vi "Insight_Reduce_Data.vi"(6 "DV Threshold":dbl=0.5, 7 "Data Valid Type":enum16{"Software DV", "Hardware DV"}(ring), 8 "error in (no error)":errorcluster, 9 "Data Valid Data":dbl[](array[numeric]), 10 "Indices of Invalid Data":u32[](array[numeric]), 11 "Raw Data":dbl[](array[numeric])) -> (0 "error out":errorcluster, 3 "Processed Data":dbl[](array[numeric]))   [LabVIEW 2011]
doc: "This VI takes Raw data and the indices of invalid measurements and reduces it to Processed Data with only valid data.\n\nYou can reduce the data using either a \"Software Data Valid\" - a vector of the invalid points - or a \"Hardware Data Valid\" - which is a vector acquired simultaneous with the Raw Data. Use the Enum to select which type you are using and provide either the \"Indices of Invalid Data\" fot \"Software Data Valid\", or the \"Data Valid Data\" and \"DV Threshold\" for \"Hardware Data Valid\"."
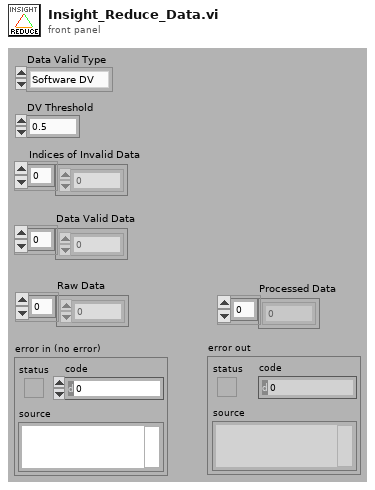
[diagram p1: front panel]
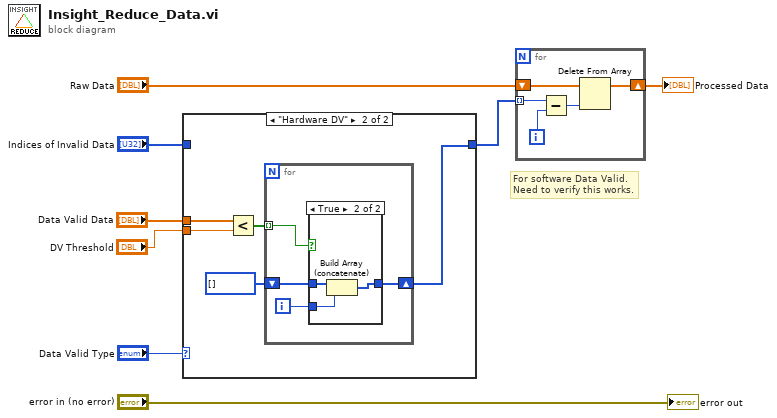
[diagram p0: block diagram]
diagram:
  # "For software Data Valid.\nNeed to verify this works."
  n1 = case shown="\"Hardware DV\"" "Data Valid Type" {
    tunnel: [w9 w13] -> w8
    tunnel: "Data Valid Data" -> [_ w11]
    tunnel: "DV Threshold" -> [_ w10]
    tunnel: "Indices of Invalid Data" -> [w9 _]
    frame "Software DV", Default {
    }
    frame "Hardware DV" {
      n2 = Less?(x=w11, y=w10) -> (x < y?=w12:bool[])
      n3 = for {
        shift-right: [w18] -> w13
        shift-left: i32[] [] -> [w16]
        tunnel: w12 -> [w15] mode=indexing
        i -> [w17]
        n4 = case shown="True" w15 {
          tunnel: [w19 w22] -> w18
          tunnel: w17 -> [_ w21]
          tunnel: w16 -> [w19 w20]
          frame False {
          }
          frame True {
            n5 = Build Array (concatenate)(w20, w21) -> (w22:i32[])
          }
        }
      }
    }
  }
  n6 = for {
    tunnel: w8 -> [w25] mode=indexing
    shift-right: [w26] -> w7
    shift-left: "Raw Data" -> [w27]
    i -> [w23]
    n7 = Subtract(x=w25, y=w23) -> (x-y=w24:u32)
    n8 = Delete From Array(array=w27, index=w24) -> (array with subset deleted=w26:dbl[])  [unwired: 1 in, 1 out]
  }
  "Processed Data" <- w7
  "error out" <- "error in (no error)"
